vi "TX OOB Test Cases.vi"() -> (0 "error out":errorcluster, 2 "status":string, 3 "pass":bool)   [LabVIEW 2021]
uses:
  <vilib>/CIF Foundation/CIF Out of Band Commands/CIFOutOfBand.lvclass
  OOB_Tx/TemplateOOB_Tx.lvclass
  OOB_Tx/Typedef/OOB Commands.ctl
  OOB_Tx/Typedef/Main to gRPC Command Data.ctl
  C:/Program Files/National Instruments/LabVIEW 2021/vi.lib/CIF Foundation/CIF Out of Band Commands/CIFOutOfBand.lvclass
  D:/dev/Plugins/Template/OOB/OOB_Tx/TemplateOOB_Tx.lvclass
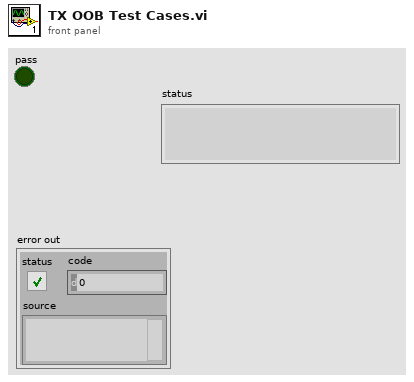
[diagram p1: front panel]
types:
  T1 = typedef "TemplateOOB_Tx.lvclass/Main to gRPC Command Data.ctl" = cluster{"Cmd 1 Data -> gRPC":i32}
  T2 = typedef "TemplateOOB_Tx.lvclass/OOB Commands.ctl" = enum8{"Command 1"}
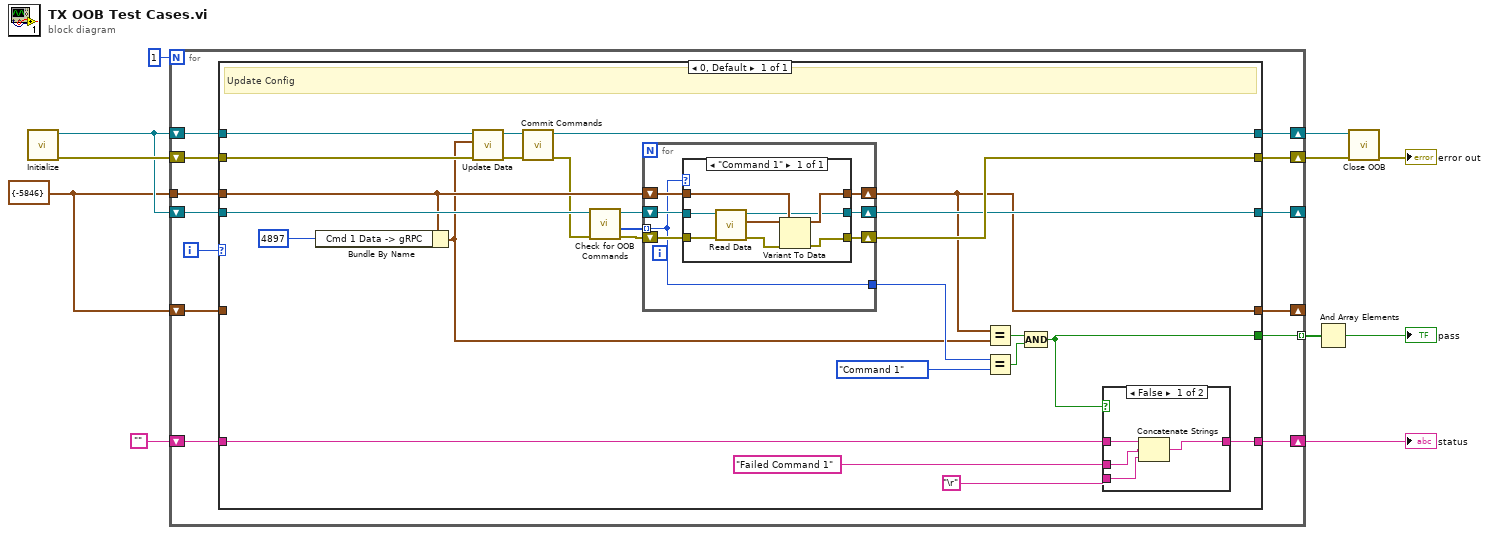
[diagram p0: block diagram]
diagram:
  w1 = T1 {"Cmd 1 Data -> gRPC"=-5846} ("Data")
  n1 = call "Initialize.vi"() -> ("error out"=w3:errorcluster, "CutomOOB_Tx out"=w2:refnum<class "TemplateOOB_Tx.lvclass">)  [unwired: 10 in]
  n2 = for {
    N: 1 -> [_]
    tunnel: [w24] -> w9 mode=indexing
    tunnel: w1 -> [w22]
    shift-right: [w21] -> w10
    shift-left: w3 -> [w23]
    shift-right: [w12] -> w11
    shift-left: w2 -> [w13]
    shift-right: [w18] -> _
    shift-left: w2 -> [w19]
    shift-right: [w17] -> _
    shift-left: w1 -> [w16]
    shift-right: [w14] -> w6
    shift-left: "" -> [w15]
    i -> [w20]
    n3 = case shown="0, Default" w20 {
      tunnel: [w37] -> w24
      tunnel: w23 -> [w34]
      tunnel: w22 -> [w33]
      tunnel: w13 -> [w31]
      tunnel: [w49] -> w21
      tunnel: [w25] -> w12
      tunnel: w19 -> [w43]
      tunnel: [w48] -> w18
      tunnel: [w32] -> w17
      tunnel: w16 -> [_]
      tunnel: w15 -> [w47]
      tunnel: [w46] -> w14
      frame 0, Default {
        # "Update Config"
        n4 = Bundle By Name(cluster=w33, "Cmd 1 Data -> gRPC"=4897 ("Numeric")) -> (w29:T1)
        n5 = call "Update Data.vi"("error in"=w34, "Data"=w29, "CutomOOB_Tx in"=w31) -> ("error out"=w27:errorcluster, "CutomOOB_Tx out"=w28:refnum<class "TemplateOOB_Tx.lvclass">)  [unwired: 7 in]
        n6 = call <vilib>:"Commit Commands.vi"("error in"=w27, "OOB in"=w28) -> ("error out"=w26:errorcluster, "OOB out"=w25:refnum<class "TemplateOOB_Tx.lvclass">)  [unwired: 8 in]
        n7 = call "Check for OOB Commands.vi"("error in (no error)"=w26, "CutomOOB_Tx in"=w43) -> ("error out"=w42:errorcluster, "Commands"=w40:T2[], "CutomOOB_Tx out"=w41:refnum<class "TemplateOOB_Tx.lvclass">)  [unwired: 6 in, 1 out]
        n8 = for {
          tunnel: w40 -> [w50] mode=indexing
          shift-right: [w51] -> w32
          shift-left: w33 -> [w56]
          shift-right: [w55] -> w49
          shift-left: w42 -> [w53]
          shift-right: [w54] -> w48
          shift-left: w41 -> [w52]
          tunnel: [w50] -> w36
          n9 = case shown="\"Command 1\"" w50 {
            tunnel: w52 -> [w60]
            tunnel: w53 -> [w61]
            tunnel: [w59] -> w54
            tunnel: w56 -> [w64]
            tunnel: [w63] -> w55
            tunnel: [w62] -> w51
            frame "Command 1" {
              n10 = call "Read Data.vi"("error in"=w61, "CutomOOB_Tx in"=w60) -> ("error out"=w57:errorcluster, "Data"=w58:T1, "CutomOOB_Tx out"=w59:refnum<class "TemplateOOB_Tx.lvclass">)  [unwired: 7 in]
              n11 = Variant To Data(error in=w57, type=w64, Variant=w58) -> (data=w62:T1, error out=w63:errorcluster)
            }
          }
        }
        n12 = Equal?(x=w32, y=w29) -> (x = y?=w39:bool)
        n13 = Equal?(x=w36, y=OOB_Commands."Command 1") -> (x = y?=w38:bool)
        n14 = Compound Arithmetic op=AND(w39, w38) -> (w37:bool)
        n15 = case shown="False" w37 {
          tunnel: w47 -> [w68 w69]
          tunnel: [w65 w69] -> w46
          tunnel: "Failed Command 1" -> [w67 _]
          tunnel: "\r" -> [w66 _]
          frame False {
            n16 = Concatenate Strings(w68, w67, w66) -> (w65:string)
          }
          frame True {
          }
        }
      }
    }
  }
  "status" <- w6
  n17 = And Array Elements(Boolean array=w9) -> (logical AND=→"pass":bool)
  n18 = call <vilib>:"Close OOB.vi"("error in"=w10, "OOB in"=w11) -> ("error out"=→"error out":errorcluster)  [unwired: 9 in]
